vi "CreateEvent_Item_OnCommand.vi"(10 "Command ID":string, 11 "Object":T1) -> ()   [LabVIEW 2014]
doc: "OnCommand\n\n\nInputs:\n---------------------\n- Command ID : String; \n- Object : U64; \n\nOutputs:\n---------------------\n\n\n----------------------------------------------\n6/8/2018 jcm\nZühlke Engineering AG\nCH-8952 Schlieren\nwww.zuehlke.com"
uses:
  <resource>/Framework/Providers/API/ItemRef.ctl
panel:
  out "error out":errorcluster
  in  "error in":errorcluster
  # "Connector Pane"
  # "Locals"
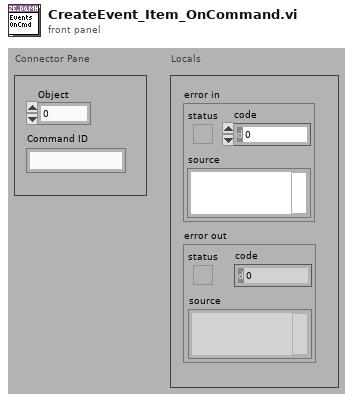
[diagram p1: front panel]
types:
  T1 = typedef "ItemRef.ctl" = u64
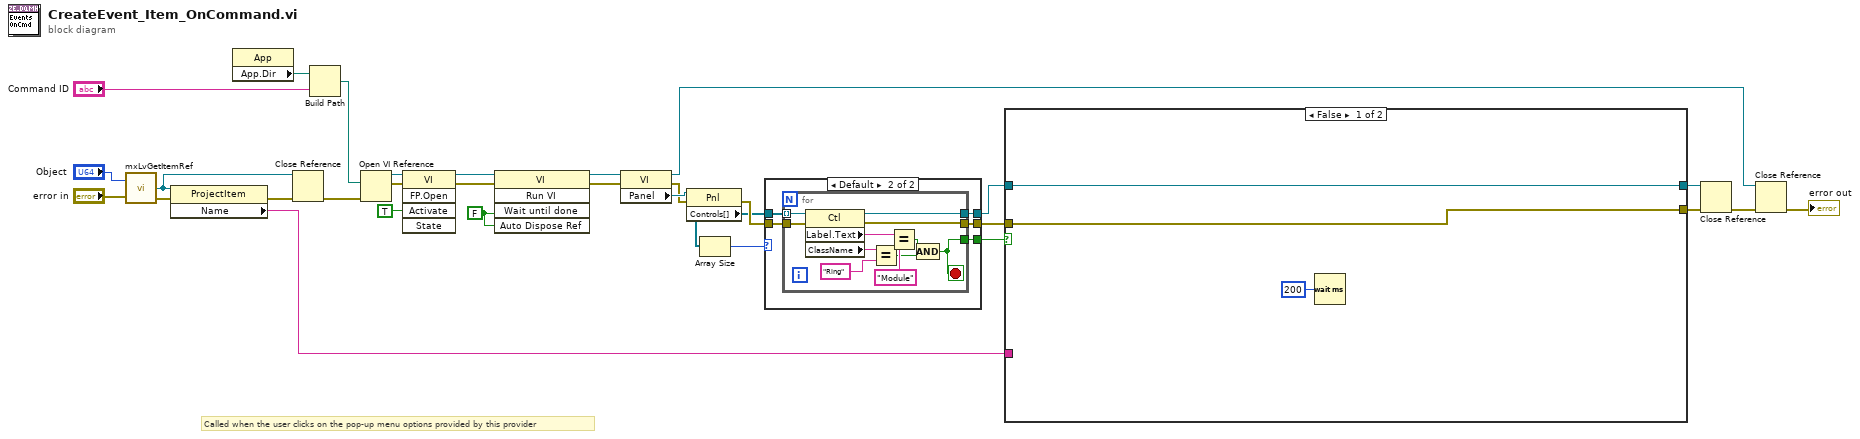
[diagram p0: block diagram]
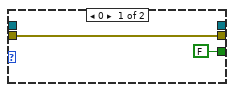
[diagram p2: hidden frame]
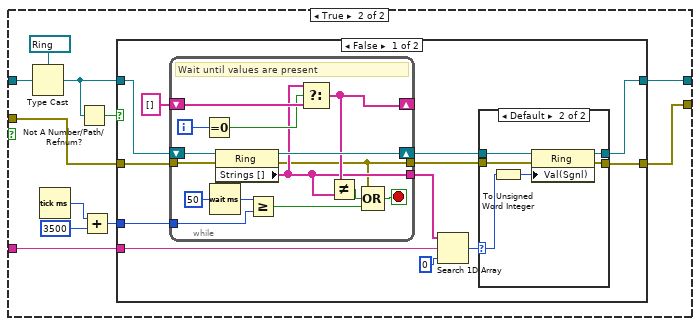
[diagram p3: hidden frame]
diagram:
  w13 = FALSE ("Wait Until Done")
  # "Called when the user clicks on the pop-up menu options provided by this provider"
  n1 = call <resource>:"mxLvGetItemRef.vi"("Item"="Object", "error in"="error in") -> ("Item Refnum"=w18:refnum<vi>, "error out"=w20:errorcluster)  [unwired: 1 out]
  n2 = property class="ProjectItem"(reference=w18, error in=w20) -> (error out=w19:errorcluster, "Name"=w17:string)  [unwired: 1 out]
  n3 = property class="App"() -> ("App.Dir"=w30:path)  [unwired: 2 in, 2 out]
  n4 = Close Reference(reference=w18, error in (no error)=w19) -> (error out=w23:errorcluster)
  n5 = Build Path(base path=w30, name or relative path="Command ID") -> (appended path=w31:path)
  n6 = Open VI Reference(vi path=w31, error in (no error)=w23) -> (vi reference=w28:refnum<vi>, error out=w27:errorcluster)  [unwired: 4 in]
  n7 = invoke class="VI" method="FP.Open"(reference=w28, error in=w27, "Activate"=TRUE ("Activate?")) -> (reference out=w26:refnum<vi>, error out=w25:errorcluster)  [unwired: 2 in, 3 out]
  n8 = invoke class="VI" method="Run VI"(reference=w26, error in=w25, "Wait until done"=w13, "Auto Dispose Ref"=w13) -> (reference out=w11:refnum<vi>, error out=w12:errorcluster)  [unwired: 1 in, 3 out]
  n9 = property class="VI"(reference=w11, error in=w12) -> (reference out=w16:refnum<vi>, error out=w6:errorcluster, "Panel"=w7:refnum<vi>)
  n10 = property class="Pnl"(reference=w7, error in=w6) -> (error out=w5:errorcluster, "Controls[]"=w4:refnum<vi>[])  [unwired: 1 out]
  n11 = Array Size(array=w4) -> (size(s)=w3:i32)
  n12 = case shown="Default" w3 {
    tunnel: [_ w38] -> w1
    tunnel: [FALSE w37] -> w14
    tunnel: w5 -> [w33 w36]
    tunnel: [w33 w35] -> w2
    tunnel: w4 -> [_ w34]
    frame 0 {
    }
    frame Default {
      n13 = for {
        tunnel: w34 -> [w49] mode=indexing
        tunnel: [w48] -> w38
        tunnel: [w39] -> w37
        tunnel: w36 -> [w45]
        tunnel: [w44] -> w35
        stop <- w39 stop-if-true
        n14 = property class="Ctl"(reference=w49, error in=w45) -> (reference out=w48:refnum<vi>, error out=w44:errorcluster, "Label.Text"=w47:string, "ClassName"=w43:string)
        n15 = Equal?(x=w43, y="Ring" ("Class Name")) -> (x = y?=w40:bool)
        n16 = Equal?(x=w47, y="Module" ("Control Name")) -> (x = y?=w41:bool)
        n17 = Compound Arithmetic op=AND(w41, w40) -> (w39:bool)
      }
    }
  }
  n18 = case shown="False" w14 {
    tunnel: w1 -> [w51 w63]
    tunnel: w2 -> [w52 w61]
    tunnel: [w52 w53] -> w10
    tunnel: w17 -> [_ w60]
    tunnel: [w51 w57] -> w8
    frame False {
      n19 = Wait (ms)(milliseconds to wait=u32 200) -> ()  [unwired: 1 out]
    }
    frame True {
      n20 = Type Cast(type=refnum<vi> refnum ("Module"), x=w63) -> (*(type *) &x=w59:refnum<vi>)
      n21 = Tick Count (ms)() -> (millisecond timer value=w56:u32)
      n22 = Not A Number/Path/Refnum?(number/path/refnum=w59) -> (NaN/Path/Refnum?=w58:bool)
      n23 = Add(x=w56, y=u32 3500) -> (x+y=w54:u32)
      n24 = case shown="False" w58 {
        tunnel: w61 -> [w74 w99]
        tunnel: w60 -> [w71 _]
        tunnel: [w69 w100] -> w57
        tunnel: w59 -> [w68 w100]
        tunnel: w54 -> [w67 _]
        tunnel: [w65 w99] -> w53
        frame False {
          n25 = while {
            tunnel: [w77] -> w72
            shift-right: [w89] -> w70
            shift-left: w68 -> [w88]
            tunnel: w74 -> [w90]
            tunnel: [w76] -> w66
            tunnel: w67 -> [w87]
            shift-right: [w78] -> _
            shift-left: string[] [] ("Strings []") -> [w82]
            i -> [w81]
            stop <- w85 stop-if-true
            # "Wait until values are present"
            n26 = Equal To 0?(x=w81) -> (x = 0?=w80:bool)
            n27 = Wait (ms)(milliseconds to wait=u32 50) -> (millisecond timer value=w84:u32)
            n28 = property class="Ring"(reference=w88, error in=w90) -> (reference out=w89:refnum<vi>, error out=w76:errorcluster, "Strings []"=w77:string[])
            n29 = Greater Or Equal?(x=w84, y=w87) -> (x >= y?=w86:bool)
            n30 = Select(t=w77, s=w80, f=w82) -> (s? t:f=w78:string[])
            n31 = Not Equal?(x=w78, y=w77) -> (x != y?=w79:bool)
            n32 = Compound Arithmetic op=OR(w76, w79, w86) -> (w85:bool)
          }
          n33 = Search 1D Array(1D array=w72, element=w71, start index (0)=0) -> (index of element=w73:i32)
          n34 = case shown="Default" w73 {
            selector: w73 -> [_ w98]
            tunnel: w70 -> [w92 w97]
            tunnel: [w92 w95] -> w69
            tunnel: w66 -> [w91 w94]
            tunnel: [w91 w93] -> w65
            frame -1 {
            }
            frame Default {
              n35 = To Unsigned Word Integer(number=w98) -> (unsigned 16bit integer=w96:u16)
              n36 = property class="Ring"(reference=w97, error in=w94, "Val(Sgnl)"=w96) -> (reference out=w95:refnum<vi>, error out=w93:errorcluster)
            }
          }
        }
        frame True {
        }
      }
    }
  }
  n37 = Close Reference(reference=w8, error in (no error)=w10) -> (error out=w9:errorcluster)
  n38 = Close Reference(reference=w16, error in (no error)=w9) -> (error out=→"error out":errorcluster)
